vi "set BK9129B voltages x3.vi"(0 "voltage in 1 (V)":dbl format="%.2f", 1 "voltage in 2 (V)":dbl format="%.2f", 2 "voltage in 3 (V)":dbl format="%.2f", 3 "error in":errorcluster, 4 "VISA in":refnum<visa-resource-name>="GPIB0::12::INSTR") -> (5 "VISA out":refnum<visa-resource-name>="GPIB0::12::INSTR", 6 "error out":errorcluster)   [LabVIEW 2020]
panel:
  out "output string":string
  # "inputs"
  # "outputs"
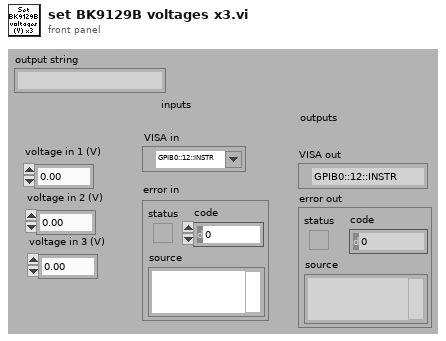
[diagram p1: front panel]
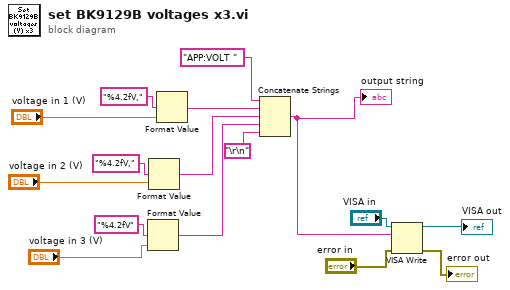
[diagram p0: block diagram]
diagram:
  n1 = Format Value(format string="%4.2fV" ("string (\"\")"), value (0)="voltage in 3 (V)") -> (output string=w10:string)  [unwired: 1 in]
  n2 = Format Value(format string="%4.2fV," ("string (\"\")"), value (0)="voltage in 2 (V)") -> (output string=w9:string)  [unwired: 1 in]
  n3 = Format Value(format string="%4.2fV," ("string (\"\")"), value (0)="voltage in 1 (V)") -> (output string=w8:string)  [unwired: 1 in]
  n4 = Concatenate Strings("APP:VOLT " ("format string"), w8, w9, w10, "\r\n") -> (w5:string)
  "output string" <- w5
  n5 = VISA Write(VISA resource name="VISA in", write buffer=w5, error in (no error)="error in") -> (VISA resource name out=→"VISA out":refnum<visa-resource-name>, error out=→"error out":errorcluster)  [unwired: 1 out]
